vi "testSendErrorExplanation.vi"(8 "error in (no error)":errorcluster) -> (0 "error out":errorcluster)   [LabVIEW 2018]
doc: "Test the sendErrorExplanation.vi."
uses:
  src/TcpServerBase/typedef/msgTypeDef.ctl
  src/TcpServerBase/TcpServerBase.lvclass
  src/TcpServerBase/TcpServerBase.lvclass/TcpServerBase.ctl
  <vilib>/addons/_JKI Toolkits/Caraya/classes/Assert/Assert Equal Type_Variant.vi
  <vilib>/addons/_JKI Toolkits/Caraya/classes/Test/Test.lvclass
  <vilib>/addons/_JKI Toolkits/Caraya/classes/Assert/Assert.lvclass
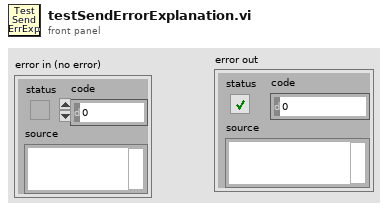
[diagram p1: front panel]
types:
  T1 = typedef "TcpServerBase.lvclass/msgTypeDef.ctl" = cluster{"msgName":string, "msgDetails":string}
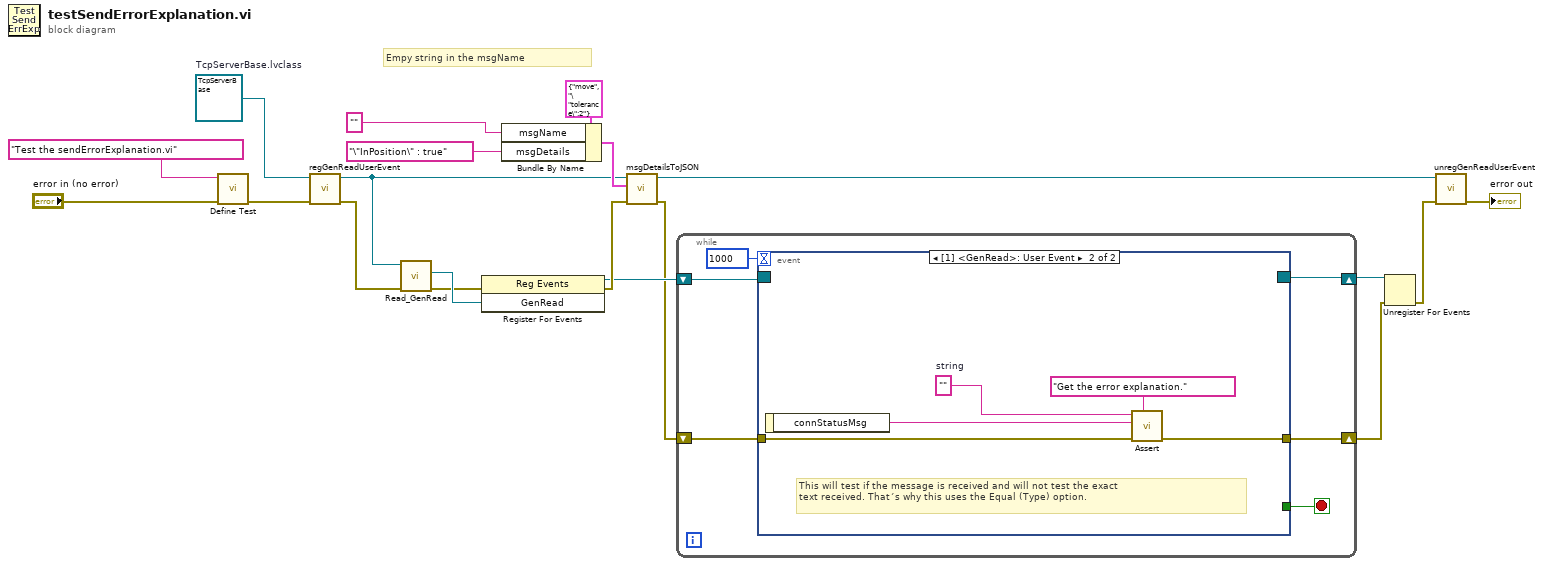
[diagram p0: block diagram]
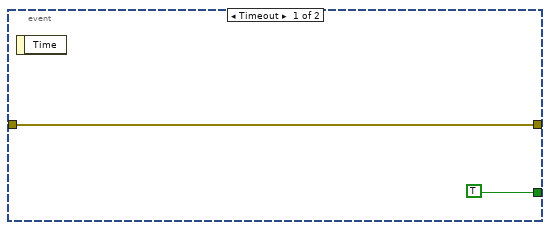
[diagram p2: hidden frame]
diagram:
  w14 = refnum<class "TcpServerBase.lvclass"> refnum  # TcpServerBase.lvclass
  # "Empy string in the msgName"
  n1 = call <vilib>:"Define Test.vi"("error in (no error)"="error in (no error)", "Label (VI Title)"="Test the sendErrorExplanation.vi") -> ("error out"=w13:errorcluster)  [unwired: 9 in]
  n2 = call "regGenReadUserEvent.vi"("error in (no error)"=w13, "TcpServerBase in"=w14) -> ("error out"=w12:errorcluster, "TcpServerBase out"=w1:refnum<class "TcpServerBase.lvclass">)  [unwired: 8 in]
  n3 = call "Read_GenRead.vi"("error in (no error)"=w12, "TcpServerBase in"=w1) -> ("error out"=w9:errorcluster, "GenRead"=w11:refnum<user-event>)  [unwired: 7 in, 1 out]
  n4 = register-events(error in=w9, w11) -> (reference out=w8:refnum<event-registration>, error out=w10:errorcluster)  [unwired: 1 in]
  n5 = Bundle By Name(cluster=T1 {"msgName"="move", "msgDetails"="\"tolerance\":2"} ("msgTypeDef"), "msgName"="" ("String"), "msgDetails"="\"InPosition\" : true" ("String")) -> (w17:T1)
  n6 = call "msgDetailsToJSON.vi"("error in (no error)"=w10, "msgData"=w17, "TcpServerBase in"=w1) -> ("error out"=w2:errorcluster, "TcpServerBase out"=w5:refnum<class "TcpServerBase.lvclass">)  [unwired: 6 in, 1 out]
  n7 = while {
    shift-right: [w23] -> w6
    shift-left: w2 -> [w21]
    shift-right: [w22] -> w7
    shift-left: w8 -> [w24]
    stop <- w25 stop-if-true
    n8 = event shown="[1] <GenRead>: User Event" {
      selector: w24 -> [_ _]
      dyn-events: [_ _] -> w22
      timeout: 1000 -> [_ _]
      tunnel: [TRUE _] -> w25
      tunnel: [w27 w32] -> w23
      tunnel: w21 -> [w27 w31]
      event Timeout {
        n9 = event-data() -> ()  [unwired: 1 in, 1 out]
      }
      event User Event {
        w29 = ""  # string
        # "This will test if the message is received and will not test the exact\ntext received. That´s why this uses the Equal (Type) option."
        n10 = event-data() -> ("connStatusMsg"=w30:string)  [unwired: 1 in]
        n11 = call-poly <vilib>:"Assert.vi"("Label"="Get the error explanation.", "error in (no error)"=w31, "Y"=w30, "X"=w29) -> ("error out"=w32:errorcluster)  [unwired: 7 in]
      }
    }
  }
  n12 = Unregister For Events(event registration refnum=w7, error in=w6) -> (error out=w4:errorcluster)
  n13 = call "unregGenReadUserEvent.vi"("error in (no error)"=w4, "tcpServerBase in"=w5) -> ("error out"=→"error out":errorcluster)  [unwired: 8 in, 1 out]
